vi "Read Temperature.vi"(8 "error in (no error)":errorcluster, 11 "Thermometer DAQmx Config in":refnum<class "Thermometer DAQmx Config.lvclass">) -> (0 "error out":errorcluster, 2 "Temperature":dbl format="%#_g °C", 3 "Thermometer DAQmx Config out":refnum<class "Thermometer DAQmx Config.lvclass">)   [LabVIEW 2023, in "Thermometer.lvlib" / "Thermometer DAQmx.lvlib" / "Thermometer DAQmx Config.lvclass"]
uses:
  Thermometer DAQmx Config.lvclass
  <vilib>/Analysis/baseanly.llb/Mean (DBL).vi
  Thermometer DAQmx Config.lvclass/Thermometer DAQmx Config.ctl
  <vilib>/Analysis/NI_AALBase.lvlib
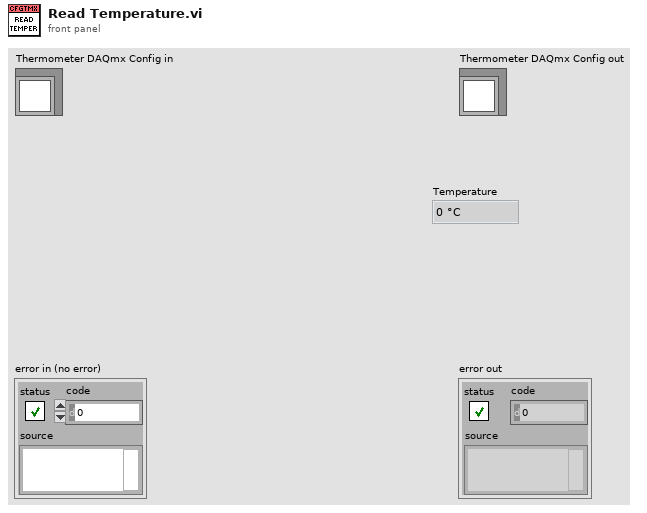
[diagram p1: front panel]
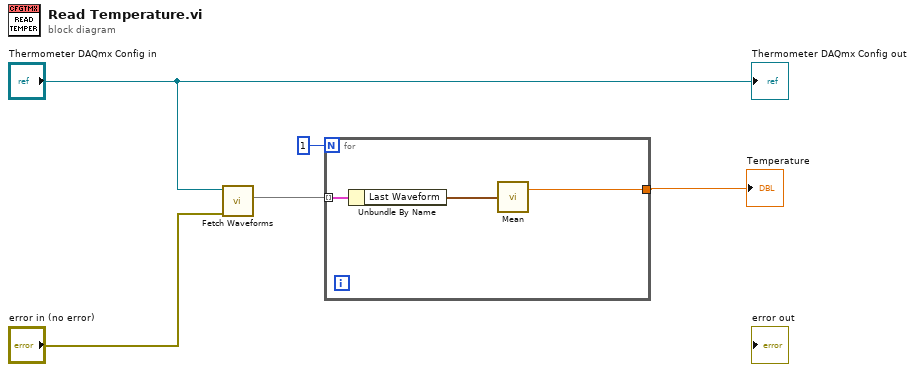
[diagram p0: block diagram]
diagram:
  n1 = call-dynamic "Fetch Waveforms.vi"("error in (no error)"="error in (no error)", "IConfigure IAI in"="Thermometer DAQmx Config in") -> ("Last Waveforms"=w2:map{u8, waveform(dbl)})  [unwired: 7 in, 2 out]
  n2 = for {
    N: 1 -> [_]
    tunnel: w2 -> [w8] mode=indexing
    tunnel: [w6] -> w1
    n3 = Unbundle By Name(w8) -> ("Last Waveform"=w7:waveform(dbl))
    n4 = call-poly <vilib>:"Mean.vi"("X"=w7) -> ("mean"=w6:dbl)  [unwired: 1 out]
  }
  "Temperature" <- w1
  "Thermometer DAQmx Config out" <- "Thermometer DAQmx Config in"
